vi "Draw Pie.vi"(4 "Legend Width":u32, 6 "Title Height":u32, 9 "State Data":T3, 10 "Draw Area Size in":T2, 11 "Margin":i16) -> (1 "mask":u8[](array[numeric]), 2 "24-bit pixmap":u32[][](array[numeric]), 3 "Pie Draw Position":cluster{"Left":u32, "Top":u32}, 5 "Pie info for Click":T1)   [LabVIEW 2018, in "PieChart.lvclass"]
uses:
  PieChart.lvclass
  <vilib>/Utility/miscctls.llb/LVBoundsTypeDef.ctl
  Pie info for Click.ctl
  <vilib>/Utility/miscctls.llb/LVFontTypeDef.ctl
  State Data.ctl
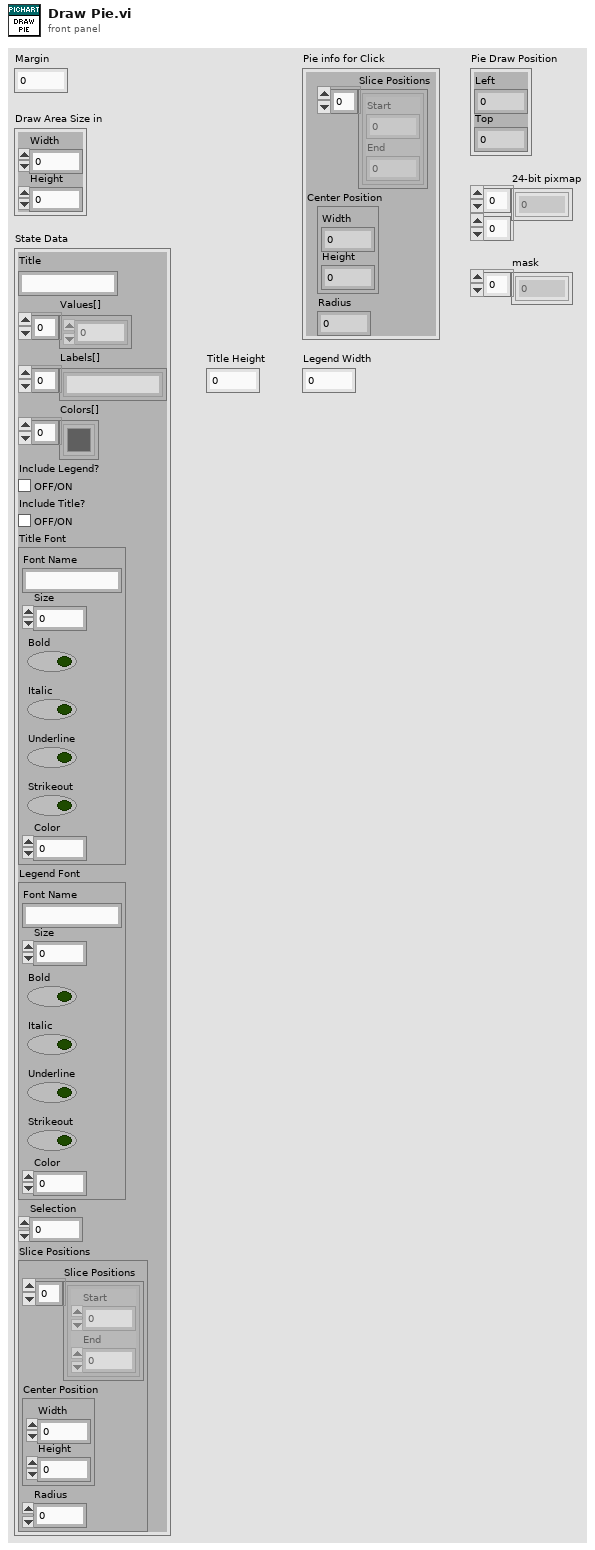
[diagram p1: front panel]
types:
  T1 = typedef "PieChart.lvclass/Pie info for Click.ctl" = cluster{"Slice Positions":cluster{"Start":i16, "End":i16}[], "Center Position":T2, "Radius":i16}
  T2 = typedef "LVBoundsTypeDef.ctl" = cluster{"Width":u32, "Height":u32}
  T3 = typedef "PieChart.lvclass/State Data.ctl" = cluster{"Title":string, "Values[]":dbl[], "Labels[]":string[], "Colors[]":u32[], "Include Legend?":bool, "Include Title?":bool, "Title Font":T4, "Legend Font":T4, "Selection":i32, "Slice Positions":T1}
  T4 = typedef "LVFontTypeDef.ctl" = cluster{"Font Name":string, "Size":u16, "Bold":bool, "Italic":bool, "Underline":bool, "Strikeout":bool, "Color":u32}
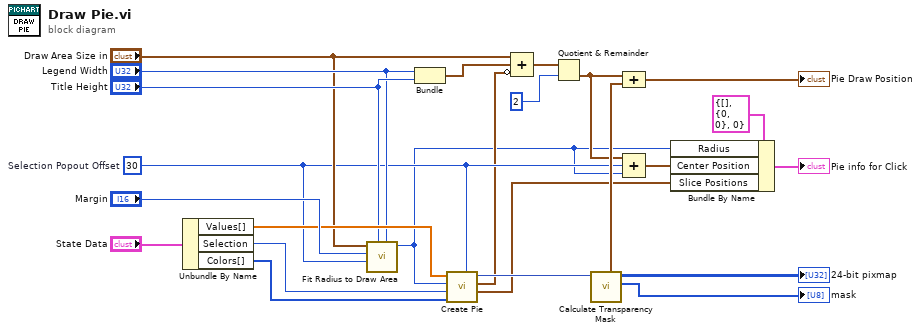
[diagram p0: block diagram]
diagram:
  w4 = i16 30  # Selection Popout Offset
  n1 = Unbundle By Name("State Data") -> ("Values[]"=w16:dbl[], "Selection"=w18:i32, "Colors[]"=w15:u32[])
  n2 = call "Fit Radius to Draw Area.vi"("Legend Width"="Legend Width", "Title Height"="Title Height", "Selection Popout Offset"=w4, "Margin"="Margin", "Draw Area Size"="Draw Area Size in") -> ("Radius"=w1:i16)  [unwired: 6 in]
  n3 = Bundle("Legend Width"="Legend Width", "Title Height"="Title Height") -> (w2:cluster{"Legend Width":u32, "Title Height":u32})  [unwired: 1 in]
  n4 = call "Create Pie.vi"("Selection Popout Offset (30)"=w4, "Colors[] (Use Default)"=w15, "Selection (-1)"=w18, "Radius"=w1, "Values[]"=w16) -> ("Slice Positions"=w7:cluster{"Start":i16, "End":i16}[], "Pie Draw Area Size"=w3:cluster{"Width":i16, "Height":i16}, "Pie out"=w17:picture)  [unwired: 4 in]
  n5 = Compound Arithmetic op=ADD("Draw Area Size in", w2, invert w3) -> (w13:T2)
  n6 = Quotient & Remainder(x=w13, y=u32 2) -> (floor(x/y)=w5:T2)  [unwired: 1 out]
  n7 = call "Calculate Transparency Mask.vi"("Picture in"=w17) -> ("mask"=→"mask":u8[], "24-bit pixmap"=→"24-bit pixmap":u32[][], "top left"=w10:cluster{"x":i16, "y":i16})  [unwired: 8 in]
  n8 = Compound Arithmetic op=ADD(w5, w10) -> (→"Pie Draw Position":T2)
  n9 = Compound Arithmetic op=ADD(w5, w4, w1) -> (w11:T2)
  n10 = Bundle By Name(cluster=T1 {"Slice Positions"=[], "Center Position"={"Width"=0, "Height"=0}, "Radius"=0}, "Radius"=w1, "Center Position"=w11, "Slice Positions"=w7) -> (→"Pie info for Click":T1)
